vi "Doğrusal Eğri.vi"() -> ()   [LabVIEW 2015]
uses:
  <vilib>/Utility/file.llb/Read Delimited Spreadsheet (DBL).vi
  <vilib>/Analysis/NI_AALPro.lvlib
panel:
  out "LİNEER EĞRİ UYDURMA":dbl[](graph)
  out "Veriler":dbl[][](array[numeric])
  in  "Okunacak Veri Adresi":path
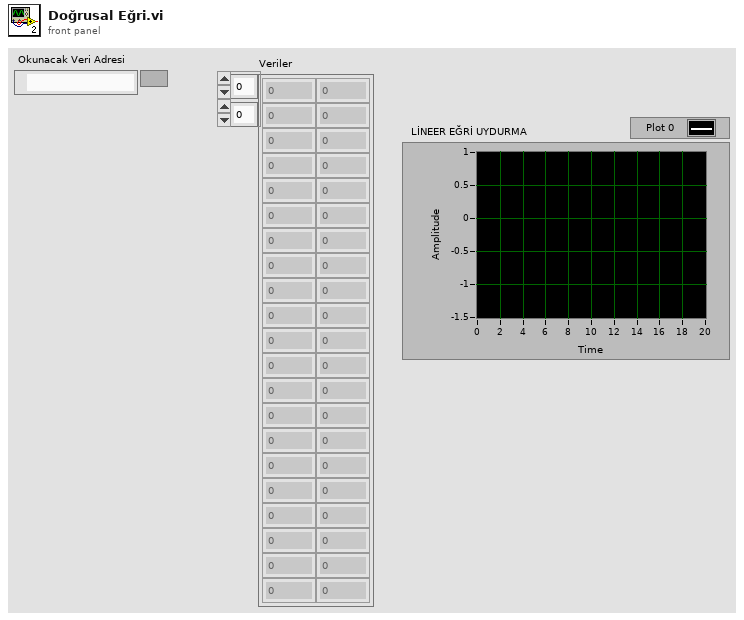
[diagram p1: front panel]
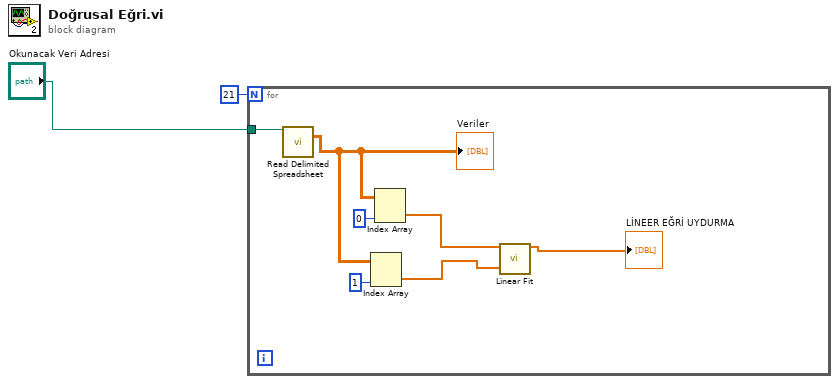
[diagram p0: block diagram]
diagram:
  n1 = for {
    N: 21 -> [_]
    tunnel: "Okunacak Veri Adresi" -> [w9]
    n2 = call-poly <vilib>:"Read Delimited Spreadsheet.vi"("file path (dialog if empty)"=w9) -> ("all rows"=w7:dbl[][])  [unwired: 9 in, 5 out]
    "Veriler" <- w7
    n3 = Index Array(array=w7, index (col)=1 ("disabled index (col)")) -> (element=w5:dbl[])  [unwired: 1 in]
    n4 = Index Array(array=w7, index (col)=0 ("disabled index (col)")) -> (element=w6:dbl[])  [unwired: 1 in]
    n5 = call <vilib>:"Linear Fit.vi"("Y"=w6, "X"=w5) -> ("Best Linear Fit"=→"LİNEER EĞRİ UYDURMA":dbl[])  [unwired: 9 in, 4 out]
  }
